vi "MeasureDetectorVoltage.vi"(10 "GPIB Address":string) -> (2 "Average Voltage":dbl)   [LabVIEW 2017]
uses:
  Linear Dichroism Controller/LD Reading.lvclass
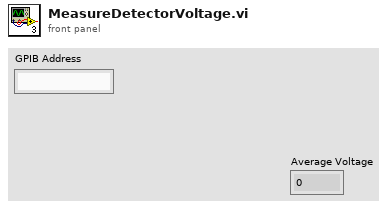
[diagram p1: front panel]
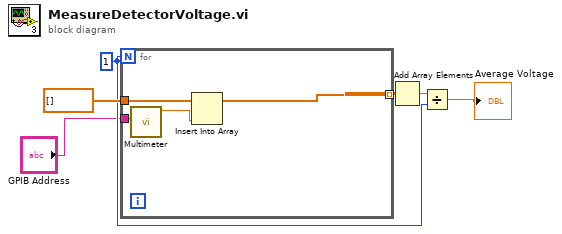
[diagram p0: block diagram]
diagram:
  w3 = 1
  n1 = for {
    N: w3 -> [_]
    tunnel: dbl[] [] ("array") -> [w10]
    tunnel: [w9] -> w5 mode=indexing
    tunnel: "GPIB Address" -> [w7]
    n2 = call "Multimeter.vi"("GPIB Address"=w7) -> ("Voltage"=w8:dbl)  [unwired: 9 in, 1 out]
    n3 = Insert Into Array(array=w10, new element=w8) -> (w9:dbl[])  [unwired: 1 in]
  }
  n4 = Add Array Elements(numeric array=w5) -> (sum=w4:dbl)
  n5 = Divide(x=w4, y=w3) -> (x/y=→"Average Voltage":dbl)
